vi "repulsive-force.vi"(8 "target pos":dbl[](array[numeric])=[338.0392150878906, -254.06089782714844] format="%#_13g", 11 "obj pos":dbl[](array[numeric])=[3750.471435546875, 295.0052490234375] format="%#_13g") -> (1 "magnitude":dbl, 3 "force":dbl[](array[numeric]))   [LabVIEW 2016]
panel:
  in  "max force":dbl=3.0 format="%#_13g"
  in  "min dist":dbl=130.0 format="%#_13g"
  in  "max dist (greater)":dbl=500.0 format="%#_13g"
  in  "power":dbl=65000.0 format="%#_13g"
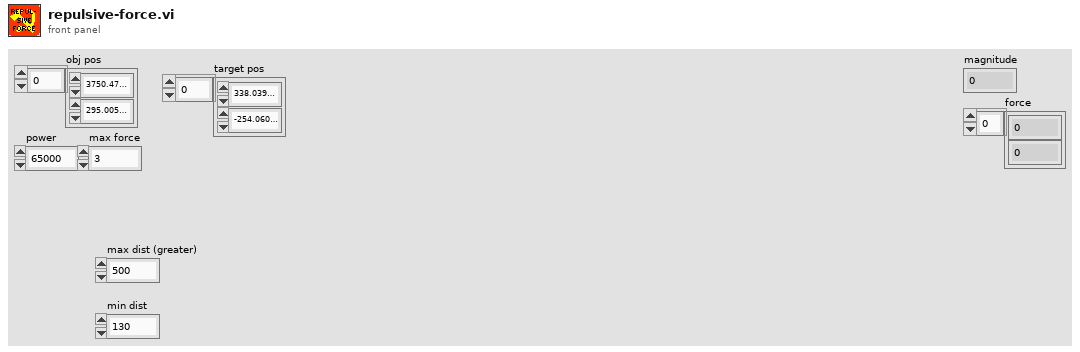
[diagram p1: front panel]
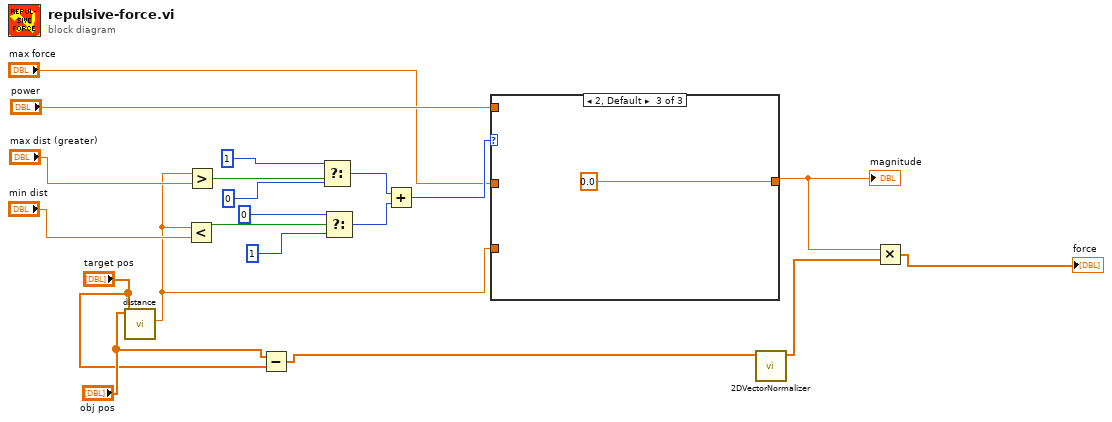
[diagram p0: block diagram]
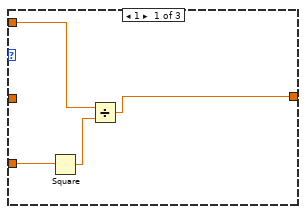
[diagram p2: hidden frame]
diagram:
  n1 = call "distance.vi"("target pos"="target pos", "obj pos"="obj pos") -> ("sqrt(x)"=w9:dbl)  [unwired: 9 in]
  n2 = Less?(x=w9, y="min dist") -> (x < y?=w14:bool)
  n3 = Greater?(x=w9, y="max dist (greater)") -> (0:w13:bool)
  n4 = Subtract(x="obj pos", y="target pos") -> (x-y=w3:dbl[])
  n5 = Select(t=1, s=w13, f=0) -> (s? t:f=w12:i32)
  n6 = Select(t=0, s=w14, f=1) -> (s? t:f=w11:i32)
  n7 = Add(x=w12, y=w11) -> (x+y=w10:i32)
  n8 = case shown="2, Default" w10 {
    tunnel: w9 -> [w24 _ _]
    tunnel: "power" -> [w22 _ _]
    tunnel: [w21 w25 0.0 ("max force")] -> w4
    tunnel: "max force" -> [_ w25 _]
    frame 1 {
      n9 = Square(x=w24) -> (x^2=w23:dbl)
      n10 = Divide(x=w22, y=w23) -> (x/y=w21:dbl)
    }
    frame 0 {
    }
    frame 2, Default {
    }
  }
  "magnitude" <- w4
  n11 = call "2DVectorNormalizer.vi"("2D vector"=w3) -> ("2D vector 2"=w2:dbl[])  [unwired: 10 in]
  n12 = Multiply(x=w4, y=w2) -> (x*y=→"force":dbl[])
